vi "Demo v3_QL.vi"() -> ()   [LabVIEW 2013]
panel:
  out "Iteration":i32
  out "h":i32
  out "w":i32
  out "Q":dbl[][](array[numeric])
  in  "Slow":bool
  out "sum":dbl
  in  "Reset Game":bool
  in  "Reset Q":bool
  in  "stop":bool
  out "JUMP?":bool
  out "SCORE":i32
  out "FAIL!":bool
  in  "a":dbl=-0.3
  in  "Jump speed":dbl=3.0
  out "Picture":i32[][](graph)
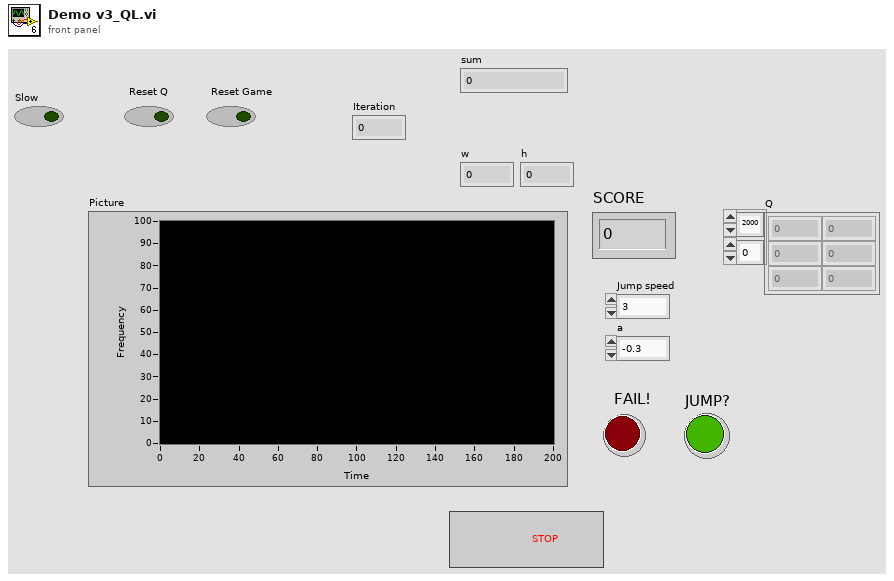
[diagram p1: front panel]
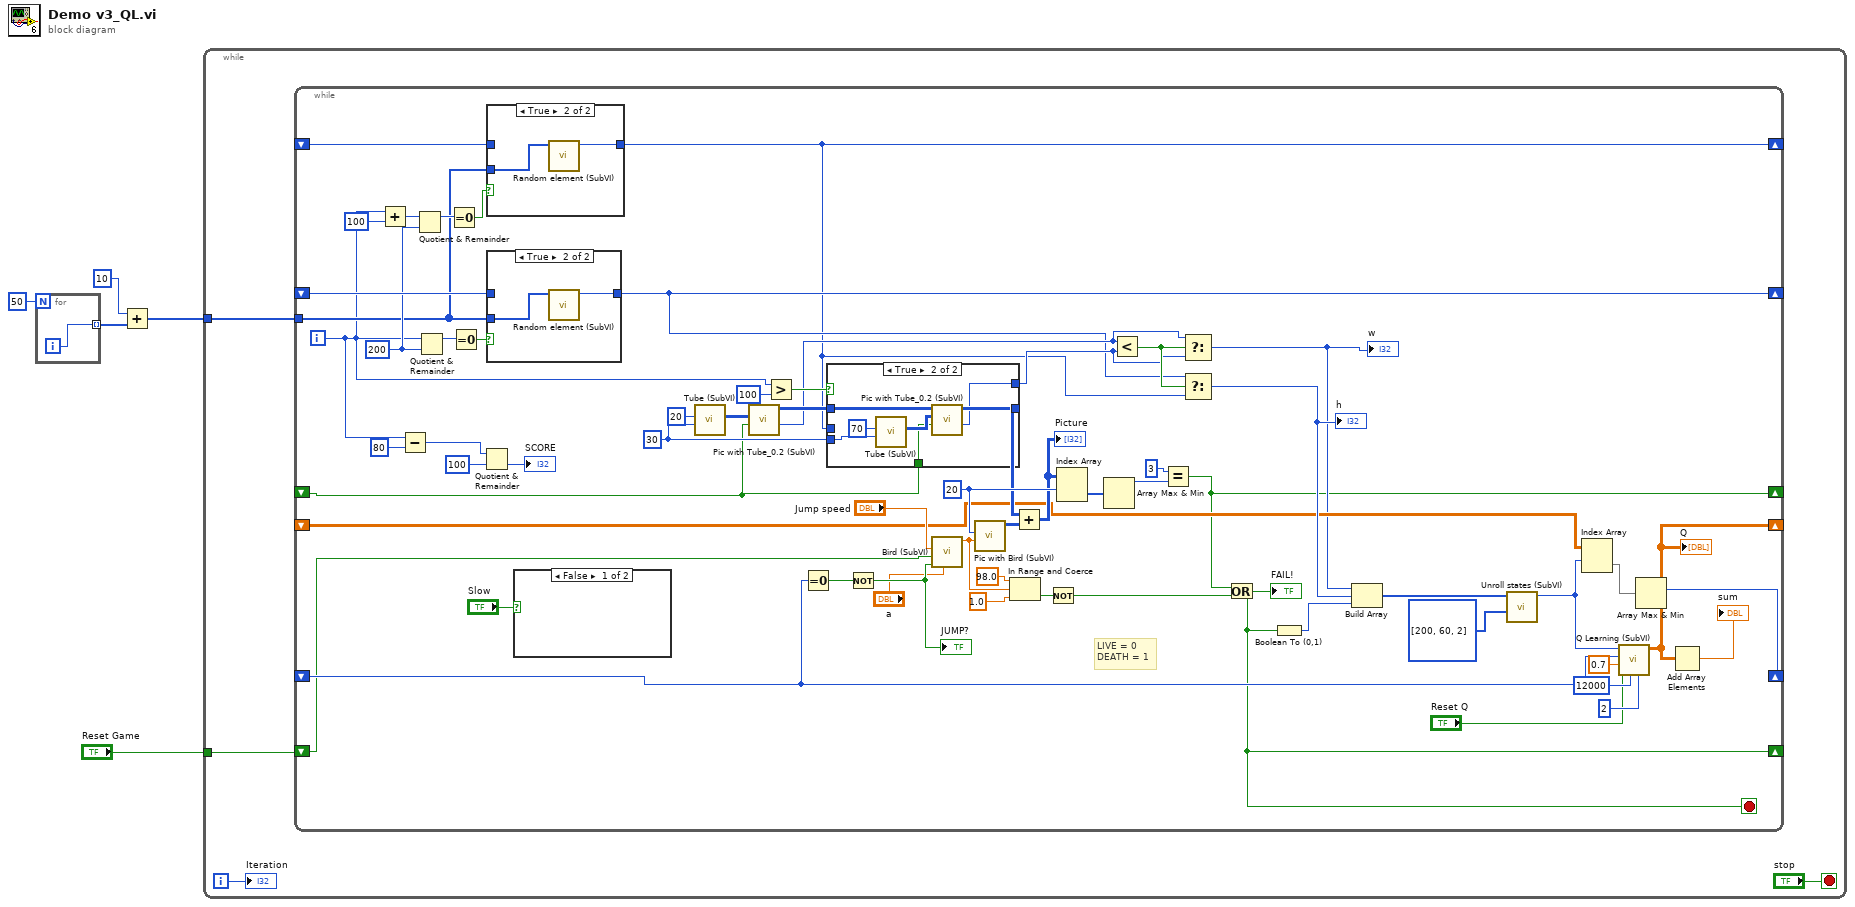
[diagram p0: block diagram]
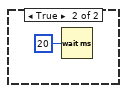
[diagram p2: hidden frame]
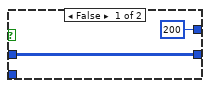
[diagram p5: hidden frame]
diagram:
  n1 = for {
    N: 50 -> [_]
    tunnel: [w6] -> w4 mode=indexing
    i -> [w6]
  }
  n2 = Add(x=10, y=w4) -> (x+y=w2:i32[])
  n3 = while {
    tunnel: w2 -> [w10]
    tunnel: "Reset Game" -> [w8]
    i -> [w7]
    stop <- "stop" stop-if-true
    n4 = while {
      tunnel: w10 -> [w46]
      shift-right: [w32] -> _
      shift-left: _ -> [w53]
      shift-right: [w31] -> _
      shift-left: _ -> [w47]
      shift-right: [w21] -> _
      shift-left: w8 -> [w14]
      shift-right: [w18] -> _
      shift-left: _ -> [w26]
      shift-right: [w23] -> _
      shift-left: _ -> [w22]
      shift-right: [w12] -> _
      shift-left: _ -> [w11]
      i -> [w43]
      stop <- w21 stop-if-true
      w49 = 200 ("y")
      w59 = 20 ("X position")
      w67 = 30 ("Gap height (30)")
      # "LIVE = 0\nDEATH = 1"
      n5 = Add(x=w43, y=100) -> (x+y=w50:i32)
      n6 = Subtract(x=w43, y=80) -> (x-y=w41:i32)
      n7 = Quotient & Remainder(x=w50, y=w49) -> (x-y*floor(x/y)=w51:i32)  [unwired: 1 out]
      n8 = Quotient & Remainder(x=w43, y=w49) -> (x-y*floor(x/y)=w55:i32)  [unwired: 1 out]
      n9 = Equal To 0?(x=w51) -> (x = 0?=w48:bool)
      n10 = Equal To 0?(x=w55) -> (x = 0?=w54:bool)
      n11 = Quotient & Remainder(x=w41, y=100) -> (floor(x/y)=→"SCORE":i32)  [unwired: 1 out]
      n12 = case shown="True" w48 {
        tunnel: [w75 w77] -> w31
        tunnel: w47 -> [w75 _]
        tunnel: w46 -> [_ w76]
        frame False {
        }
        frame True {
          n13 = call "Random element (SubVI).vi"("Array"=w76) -> ("random element"=w77:i32)  [unwired: 10 in]
        }
      }
      n14 = case shown="True" w54 {
        tunnel: [w78 w80] -> w32
        tunnel: w53 -> [w78 _]
        tunnel: w46 -> [_ w79]
        frame False {
        }
        frame True {
          n15 = call "Random element (SubVI).vi"("Array"=w79) -> ("random element"=w80:i32)  [unwired: 10 in]
        }
      }
      n16 = case shown="False" "Slow" {
        frame False {
        }
        frame True {
          n17 = Wait (ms)(milliseconds to wait=u32 20) -> ()  [unwired: 1 out]
        }
      }
      n18 = call "Tube (SubVI).vi"("Gap height (30)"=w67, "Gap low y"=20) -> ("Tube"=w71:i32[][])  [unwired: 9 in]
      n19 = call "Pic with Tube_0.2 (SubVI).vi"("Reset"=w11, "Tube"=w71) -> ("Tube X"=w34:i32, "Picture"=w70:i32[][])  [unwired: 8 in]
      n20 = Greater?(x=w43, y=100) -> (0:w68:bool)
      n21 = Equal To 0?(x=w22) -> (x = 0?=w29:bool)
      n22 = case shown="True" w68 {
        tunnel: [w82 w88] -> w58
        tunnel: w70 -> [w82 w89]
        tunnel: w67 -> [_ w86]
        tunnel: w31 -> [_ _]
        tunnel: [200 ("Tube X") w85] -> w33
        tunnel: w11 -> [_ w83]
        frame False {
        }
        frame True {
          n23 = call "Tube (SubVI).vi"("Gap height (30)"=w86, "Gap low y"=70) -> ("Tube"=w87:i32[][])  [unwired: 9 in]
          n24 = call "Pic with Tube_0.2 (SubVI).vi"("Reset"=w83, "Tube"=w87, "Picture in"=w89) -> ("Tube X"=w85:i32, "Picture"=w88:i32[][])  [unwired: 7 in]
        }
      }
      n25 = Not(x=w29) -> (.not. x?=w28:bool)
      "JUMP?" <- w28
      n26 = call "Bird (SubVI).vi"("a"="a", "Jump"=w28, "Reset"=w14, "Jump speed"="Jump speed") -> ("Position"=w66:dbl)  [unwired: 7 in]
      n27 = call "Pic with Bird (SubVI).vi"("Bird Position"=w66, "X position"=w59) -> ("Picture"=w73:i32[][])  [unwired: 9 in]
      n28 = In Range and Coerce(upper limit=98.0, x=w66, lower limit=1.0) -> (In Range?=w63:bool)  [unwired: 1 out]
      n29 = Add(x=w58, y=w73) -> (x+y=w57:i32[][])
      "Picture" <- w57
      n30 = Not(x=w63) -> (.not. x?=w56:bool)
      n31 = Index Array(array=w57, index (row)=w59) -> (element=w62:i32[])  [unwired: 1 in]
      n32 = Array Max & Min(array=w62) -> (max value=w61:i32)  [unwired: 3 out]
      n33 = Less?(x=w34, y=w33) -> (x < y?=w35:bool)
      n34 = Equal?(x=3 ("y"), y=w61) -> (x = y?=w12:bool)
      n35 = Select(t=w34, s=w35, f=w33) -> (s? t:f=w13:i32)
      "w" <- w13
      n36 = Select(t=w32, s=w35, f=w31) -> (s? t:f=w30:i32)
      "h" <- w30
      n37 = Or(x=w12, y=w56) -> (x .or. y?=w21:bool)
      "FAIL!" <- w21
      n38 = Boolean To (0,1)(Boolean=w21) -> (0, 1=w20:i16)
      n39 = Build Array(w13, w30, w20) -> (w36:i32[])
      n40 = call "Unroll states (SubVI).vi"("# each state"=i32[] [200, 60, 2], "State array"=w36) -> ("Unrolled state"=w25:i32)  [unwired: 9 in]
      n41 = Index Array(array=w26, index (row)=w25) -> (element=w24:dbl[])  [unwired: 1 in]
      n42 = call "Q Learning (SubVI).vi"("# action"=2, "# state"=12000, "Reset"="Reset Q", "Gamma"=0.7, "Action"=w22, "State"=w25) -> ("Q"=w18:dbl[][])  [unwired: 5 in]
      "Q" <- w18
      n43 = Array Max & Min(array=w24) -> (max index (indices)=w23:i32)  [unwired: 3 out]
      n44 = Add Array Elements(numeric array=w18) -> (sum=→"sum":dbl)
    }
    "Iteration" <- w7
  }
